vi "SMS FlexRIO Example_FPGA_Vanilla.vi"() -> ()   [LabVIEW 2015]
uses:
  <vilib>/Platform/TimedLoop/XDataNode/timing_clust.ctl
  <vilib>/Platform/TimedLoop/XDataNode/nitl_modes.ctl
  <vilib>/Platform/TimedLoop/XDataNode/wakeup.ctl
  <vilib>/rvi/Emulation/niFpgaSctlEmulationGetInTimedLoop.vi
  <vilib>/rvi/Emulation/niFpgaEmulationReportErrorSimple.vi
  <vilib>/rvi/Emulation/niFpgaGetClockAttributes.vi
  <vilib>/rvi/Emulation/niFpgaCriticalErrorInLSC.vi
  <vilib>/rvi/eio/common/nirviEmuTemplateMethod_errors.vi
  <vilib>/rvi/Emulation/niFpgaProcessEmulError.vi
  <instrlib>/_niInstr/Basic Elements/v1/FPGA/Private/Count Up U64.vi
  <vilib>/rvi/interface/RandomDataEmulation/niFpgaRandomDataHandleErrors.vi
  <vilib>/Platform/TimedLoop/XDataNode/XDataNode.xnode
  <vilib>/eio/EIONode/EIONode.xnode
  <vilib>/rvi/DataTransferAndStorage/Container/XNode/niFpgaContainer.xnode
  <vilib>/rvi/interface/RandomDataEmulation/nirviRandomDataFpgaReadWriteTemplate.vi
  <vilib>/Platform/TimedLoop/XDataNode/XDNodeRunTimeDep.lvlib
  <instrlib>/_niInstr/Basic Elements/v1/FPGA/niInstr Basic Elements v1 FPGA.lvlib
panel:
  out "DMA Fault":bool
  in  "Capture Enabled":bool
  out "Throughput Count":u64
  in  "Throughput Reset Period":u64
  out "Capture Count":u64
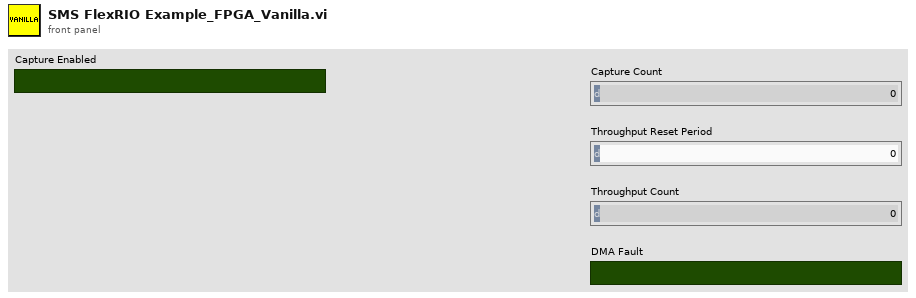
[diagram p1: front panel]
types:
  T1 = typedef "XDNodeRunTimeDep.lvlib/timing_clust.ctl" = cluster{"Expected End [f-1]":u64, "Actual End [f-1]":u64, "Finished Late? [f-1]":bool, "Expected End [i-1]":u64, "Actual End [i-1]":u64, "Finished Late? [i-1]":bool, "Expected Start [i]":u64, "Actual Start [i]":u64, "Expected Start [f]":u64, "Actual Start [f]":u64, "Source Name":string, "Structure Name":string, "Period":i64, "Deadline":i64, "Offset":i64, "Start":i64, "Priority":i32, "Timeout":i32, "Mode":T2, "Wakeup Reason":T3, "Error":errorcluster, "Source Type":string, "Secondary Source Type":string, "Global End Time":u64, "Global Start Time":u64, "Frame Duration":u64, "Iteration Duration":u64, "Assigned CPU":i32, "I/O Scan Engine Mode":u32}
  T2 = typedef "XDNodeRunTimeDep.lvlib/nitl_modes.ctl" = enum32{"No Change", "Process missed periods, maintain original phase", "Discard missed periods, maintain original phase", "Process missed periods, ignore original phase", "Discard missed periods, ignore original phase"}
  T3 = typedef "XDNodeRunTimeDep.lvlib/wakeup.ctl" = enum32{"Normal", "Aborted", "Asynchronous wakeup", "Timing source error", "Timed loop error", "Timeout"}
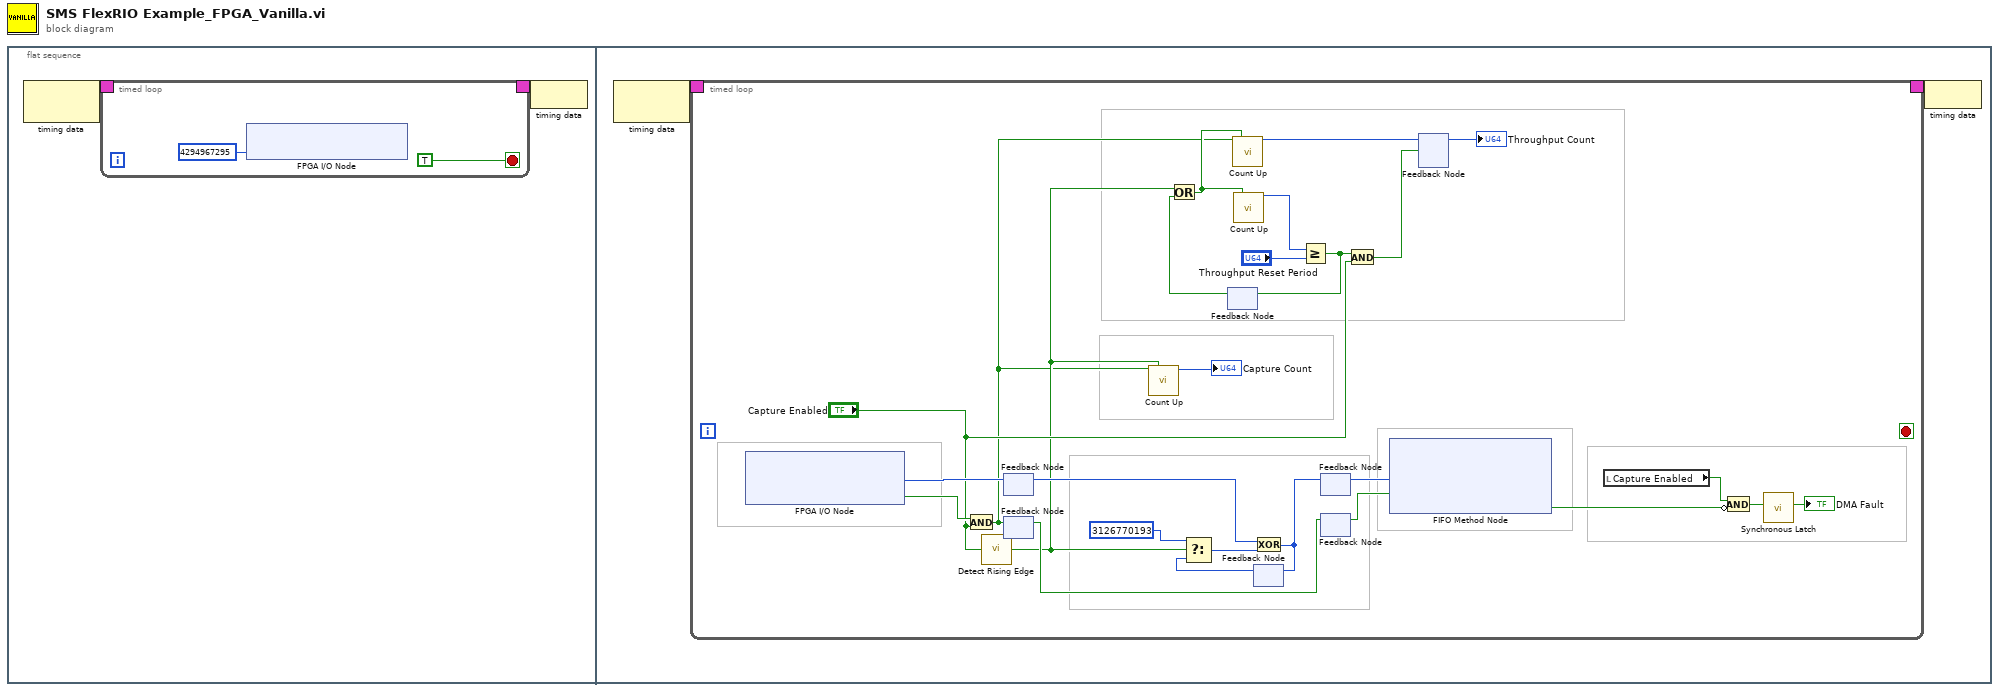
[diagram p0: block diagram]
diagram:
  n1 = flat-sequence {
    frame #0 {
      n2 = node-c288() -> (w2:T1)  [unwired: 1 in]
      n3 = timed-loop {
        timing: w2 -> [_]
        timing-out: [_] -> w1
        stop <- TRUE stop-if-true
        n4 = xnode "FPGA I/O Node"("IO Module\\SE_Data_Dir"=u32 4294967295 ("IO Module\\SE_Data_Dir")) -> ()  [unwired: 1 in, 1 out]
      }
      n5 = node-c288(w1) -> ()
    }
    frame #1 {
      n6 = node-c288() -> (w10:T1)  [unwired: 1 in]
      n7 = timed-loop {
        timing: w10 -> [_]
        timing-out: [_] -> w9
        stop <- _ stop-if-true
        n8 = xnode "FPGA I/O Node"() -> ("IO Module\\SE_Data_Rd"=w36:u32, "IO Module\\SE_PFI1_Rd"=w16:bool)  [unwired: 2 in, 2 out]
        n9 = And(x=w16, y="Capture Enabled") -> (x .and. y?=w11:bool)
        n10 = call <instrlib>:"Detect Rising Edge.vi"("signal"="Capture Enabled") -> ("edge detected"=w12:bool)  [unwired: 14 in]
        n11 = feedback-in #1(w36) -> ()
        n12 = feedback #1() -> (w19:u32)  [unwired: 1 in]
        n13 = feedback #2() -> (w15:bool)  [unwired: 1 in]
        n14 = feedback-in #2(w11) -> ()
        n15 = call-poly <instrlib>:"Count Up.vi"("increment"=w11, "reset"=w12) -> ("count out"=→"Capture Count":u64)  [unwired: 13 in]
        n16 = feedback #3() -> (w34:bool)  [unwired: 1 in]
        n17 = Or(x=w12, y=w34) -> (x .or. y?=w28:bool)
        n18 = call-poly <instrlib>:"Count Up.vi"("increment"=w11, "reset"=w28) -> ("count out"=w29:u64)  [unwired: 13 in]
        n19 = call-poly <instrlib>:"Count Up.vi"("reset"=w28) -> ("count out"=w30:u64)  [unwired: 14 in]
        n20 = feedback #4() -> (w20:u32)  [unwired: 1 in]
        n21 = Select(t=u32 3126770193, s=w12, f=w20) -> (s? t:f=w17:u32)
        n22 = Exclusive Or(1:w17, 2:w19) -> (0:w18:u32)
        n23 = feedback-in #4(w18) -> ()
        n24 = Greater Or Equal?(x=w30, y="Throughput Reset Period") -> (x >= y?=w33:bool)
        n25 = feedback-in #3(w33) -> ()
        n26 = feedback-in #5(w18) -> ()
        n27 = feedback #5() -> (w26:u32)  [unwired: 1 in]
        n28 = feedback #6() -> (w14:bool)  [unwired: 1 in]
        n29 = feedback-in #6(w15) -> ()
        n30 = And(x=w33, y="Capture Enabled") -> (x .and. y?=w27:bool)
        n31 = xnode ("FIFO Method Node")("Element"=w26, "Input Valid"=w14) -> ("Ready for Input"=w25:bool)  [unwired: 1 in, 1 out]
        n32 = feedback #7() -> (→"Throughput Count":u64)  [unwired: 1 in]
        n33 = feedback-in #7(w29, w27) -> ()
        n34 = local read "Capture Enabled"() -> (w23:bool)
        n35 = Compound Arithmetic op=AND(w23, invert w25) -> (w24:bool)
        n36 = call <instrlib>:"Synchronous Latch.vi"("set"=w24) -> ("out"=→"DMA Fault":bool)  [unwired: 10 in]
      }
      n37 = node-c288(w9) -> ()
    }
  }
